vi "Send Acyclic Frame.vi"(0 "RT Data in":T1 {"End System Handle" format="%x"; "Label Transfer Config"."Block Data Refs"."Data Reference" format="%.0x"; "Status Config"."Hardware Out Dur Reference" format="%.0x"; "Status Config"."Hardware In Dur Reference" format="%.0x"; "Status Config"."Hardware Out Count Reference" format="%.0x"; "Status Config"."Hardware In Count Reference" format="%.0x"; "Status Config"."Error Data Reference" format="%.0x"; "Hardware Output Tx Channels"."Message Settings"."Transmit Channel Data Reference" format="%.0x"; "Hardware Output Tx Channels"."Message Settings"."Queue Transmit Channel" format="%.0x"; "Hardware Output Tx Channels"."Message Settings"."Driver Data"."Num Bits" min=1 max=32; "Hardware Output Tx Channels"."Message Settings"."Block Data Refs"."Data Reference" format="%.0x"; "Hardware Output Tx Channels"."Rx Com Udp Port"."Handle" format="%08x"; "Hardware Output Tx Channels"."Tx Com Udp Port"."Handle" format="%08x"; "Hardware Input Rx Channels"."Message Settings"."Transmit Channel Data Reference" format="%.0x"; "Hardware Input Rx Channels"."Message Settings"."Queue Transmit Channel" format="%.0x"; "Hardware Input Rx Channels"."Message Settings"."Driver Data"."Num Bits" min=1 max=32; "Hardware Input Rx Channels"."Message Settings"."Block Data Refs"."Data Reference" format="%.0x"; "Hardware Input Rx Channels"."Rx Com Udp Port"."Handle" format="%08x"; "Hardware Input Rx Channels"."Tx Com Udp Port"."Handle" format="%08x"}, 9 "Device Reference in":T9 format="%.0x", 11 "error in (no error)":errorcluster, 12 "Index":i32=1) -> (4 "RT Data out":T1 {"End System Handle" format="%x"; "Label Transfer Config"."Block Data Refs"."Data Reference" format="%.0x"; "Status Config"."Hardware Out Dur Reference" format="%.0x"; "Status Config"."Hardware In Dur Reference" format="%.0x"; "Status Config"."Hardware Out Count Reference" format="%.0x"; "Status Config"."Hardware In Count Reference" format="%.0x"; "Status Config"."Error Data Reference" format="%.0x"; "Hardware Output Tx Channels"."Message Settings"."Transmit Channel Data Reference" format="%.0x"; "Hardware Output Tx Channels"."Message Settings"."Queue Transmit Channel" format="%.0x"; "Hardware Output Tx Channels"."Message Settings"."Driver Data"."Num Bits" min=1 max=32; "Hardware Output Tx Channels"."Message Settings"."Block Data Refs"."Data Reference" format="%.0x"; "Hardware Output Tx Channels"."Rx Com Udp Port"."Handle" format="%08x"; "Hardware Output Tx Channels"."Tx Com Udp Port"."Handle" format="%08x"; "Hardware Input Rx Channels"."Message Settings"."Transmit Channel Data Reference" format="%.0x"; "Hardware Input Rx Channels"."Message Settings"."Queue Transmit Channel" format="%.0x"; "Hardware Input Rx Channels"."Message Settings"."Driver Data"."Num Bits" min=1 max=32; "Hardware Input Rx Channels"."Message Settings"."Block Data Refs"."Data Reference" format="%.0x"; "Hardware Input Rx Channels"."Rx Com Udp Port"."Handle" format="%08x"; "Hardware Input Rx Channels"."Tx Com Udp Port"."Handle" format="%08x"}, 15 "error out":errorcluster)   [LabVIEW 2013, in "AIT 664 Custom Device.lvlib"]
doc: "Configure com udp queued transmit hardware output channels. These channels only send when the user sets 'Transmit' high. The Transmit channel is reset to zero after the data is sent out the AIT 664 card."
uses:
  AIT 664 Custom Device.lvlib
  <vilib>/NI Veristand/Custom Device API/Custom Device Item Ref.ctl
  RT Controls/AIT 664  - RT Data.ctl
  RT Controls/AIT 664 - RT Hardware Channel.ctl
  RT Controls/AIT 664 - RT Message Settings.ctl
  <vilib>/NI Veristand/Custom Device API/Block Data Reference.ctl
  <vilib>/NI Veristand/Custom Device API/Data Reference.ctl
  RT Controls/AIT 664 - Driver Data.ctl
  Controls and Global/Start Bit.ctl
  Controls and Global/Number of Bits.ctl
  <userlib>/ARINC 664/AIT 664 Controls/General/Message Port.ctl
  <userlib>/ARINC 664/AIT 664 Controls/General/Direction.ctl
  <userlib>/ARINC 664/AIT 664 Controls/General/Message Port Type.ctl
  System Explorer/Controls/664 - Sampling Type.ctl
  RT Controls/Status Channels Config.ctl
  RT Controls/FIFO.ctl
  RT Controls/Label Transfer Config.ctl
  <vilib>/NI Veristand/Custom Device API/Data Access Type.ctl
  <vilib>/NI Veristand/Custom Device API/Global Data Refs.vi
  <vilib>/NI Veristand/Custom Device API/Custom Device API.lvlib
  <userlib>/ARINC 664/AIT 664 API.lvlib
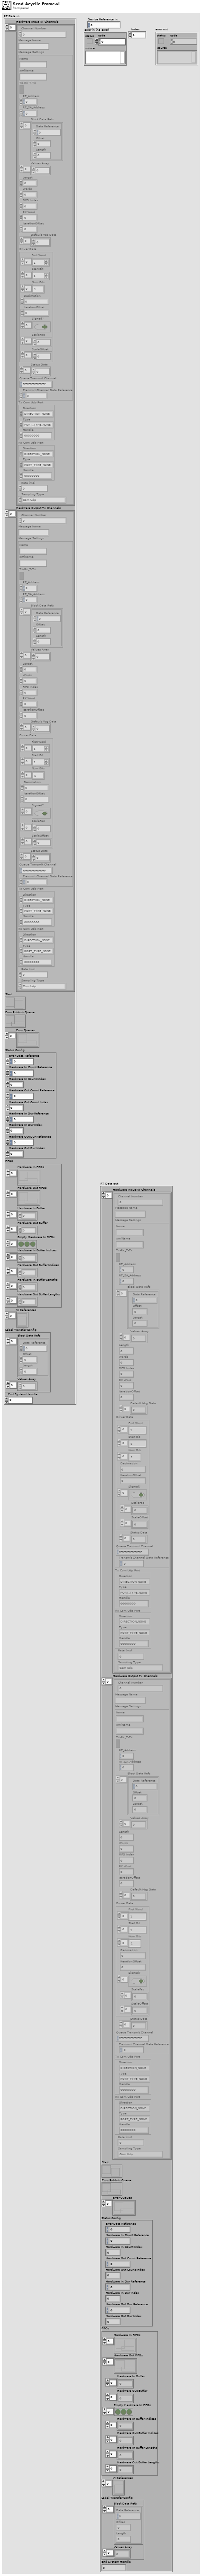
[diagram p1: front panel]
types:
  T1 = typedef "AIT 664 Custom Device.lvlib/AIT 664  - RT Data.ctl" = cluster{"Hardware Input Rx Channels":T2[], "Hardware Output Tx Channels":T2[], "Start":refnum<notifier>, "Error Publish Queue":refnum<queue>, "Error Queues":refnum<queue>[], "Status Config":T14, "FIFOs":T15, "VI References":refnum<vi>[], "Label Transfer Config":T16, "End System Handle ":u64}
  T2 = typedef "AIT 664 Custom Device.lvlib/AIT 664 - RT Hardware Channel.ctl" = cluster{"Channel Number":u16, "Message Name":string, "Message Settings":T3, "Tx Com Udp Port":T10, "Rx Com Udp Port":T10, "Rate (ms)":u32, "Sampling Type":T13}
  T3 = typedef "AIT 664 Custom Device.lvlib/AIT 664 - RT Message Settings.ctl" = cluster{"Name":string, "xmlName":string, "Tx-Rx_T-Tx":bool, "RT_Address":u8, "RT_SA_Address":u8, "Block Data Refs":T4[], "Values Array":dbl[], "Length":i32, "Words":i32, "FIFO Index":i32, "RX Word":u32, "IterationOffset":i32, "Default Msg Data":u8[], "Driver Data":T6, "Status Data":u32[], "Queue Transmit Channel":T9, "Transmit Channel Data Reference":T5}
  T4 = typedef "Custom Device API.lvlib/Block Data Reference.ctl" = cluster{"Data Reference":T5, "Offset":i32, "Length":i32}
  T5 = typedef "Custom Device API.lvlib/Data Reference.ctl" = i32
  T6 = typedef "AIT 664 Custom Device.lvlib/AIT 664 - Driver Data.ctl" = cluster{"First Word":T7[], "Start Bit":T7[], "Num Bits":T8[], "Decimation":i32, "IterationOffset":i32, "Signed?":bool[], "ScaleFac":dbl[], "ScaleOffset":dbl[]}
  T7 = typedef "AIT 664 Custom Device.lvlib/Start Bit.ctl" = i32
  T8 = typedef "AIT 664 Custom Device.lvlib/Number of Bits.ctl" = i32
  T9 = typedef "Custom Device API.lvlib/Custom Device Item Ref.ctl" = u64
  T10 = typedef "AIT 664 API.lvlib/Message Port.ctl" = cluster{"Direction":T11, "Type":T12, "Handle":u64}
  T11 = typedef "AIT 664 API.lvlib/Direction.ctl" = enum16{"DIRECTION_NONE", "DIRECTION_TX", "DIRECTION_RX"}
  T12 = typedef "AIT 664 API.lvlib/Message Port Type.ctl" = enum16{"PORT_TYPE_NONE", "COM_UDP", "SAP_UDP", "SAP_IP", "SAP_MAC", "COTS_MAC", "COTS_MAC_RAW"}
  T13 = typedef "AIT 664 Custom Device.lvlib/664 - Sampling Type.ctl" = enum16{"Com Udp", "Com Udp Queuing", "Sap Udp", "Sap Ip", "Sap Mac", "Unknown"}
  T14 = typedef "AIT 664 Custom Device.lvlib/Status Channels Config.ctl" = cluster{"Error Data Reference":T5, "Hardware In Count Reference":T5, "Hardware In Count Index":i32, "Hardware Out Count Reference":T5, "Hardware Out Count Index":i32, "Hardware In Dur Reference":T5, "Hardware In Dur Index":i32, "Hardware Out Dur Reference":T5, "Hardware Out Dur Index":i32}
  T15 = typedef "AIT 664 Custom Device.lvlib/FIFO.ctl" = cluster{"Hardware In FIFOs":refnum<k33>[], "Hardware Out FIFOs":refnum<k33>[], "Hardware In Buffer":dbl[], "Hardware Out Buffer":dbl[], "Empty Hardware In FIFOs":bool[], "Hardware In Buffer Indices":i32[], "Hardware Out Buffer Indices":i32[], "Hardware In Buffer Lengths":i32[], "Hardware Out Buffer Lengths":i32[]}
  T16 = typedef "AIT 664 Custom Device.lvlib/Label Transfer Config.ctl" = cluster{"Block Data Refs":T4[], "Values Array":dbl[]}
  T17 = typedef "Custom Device API.lvlib/Data Access Type.ctl" = enum16{"Read", "Write"}
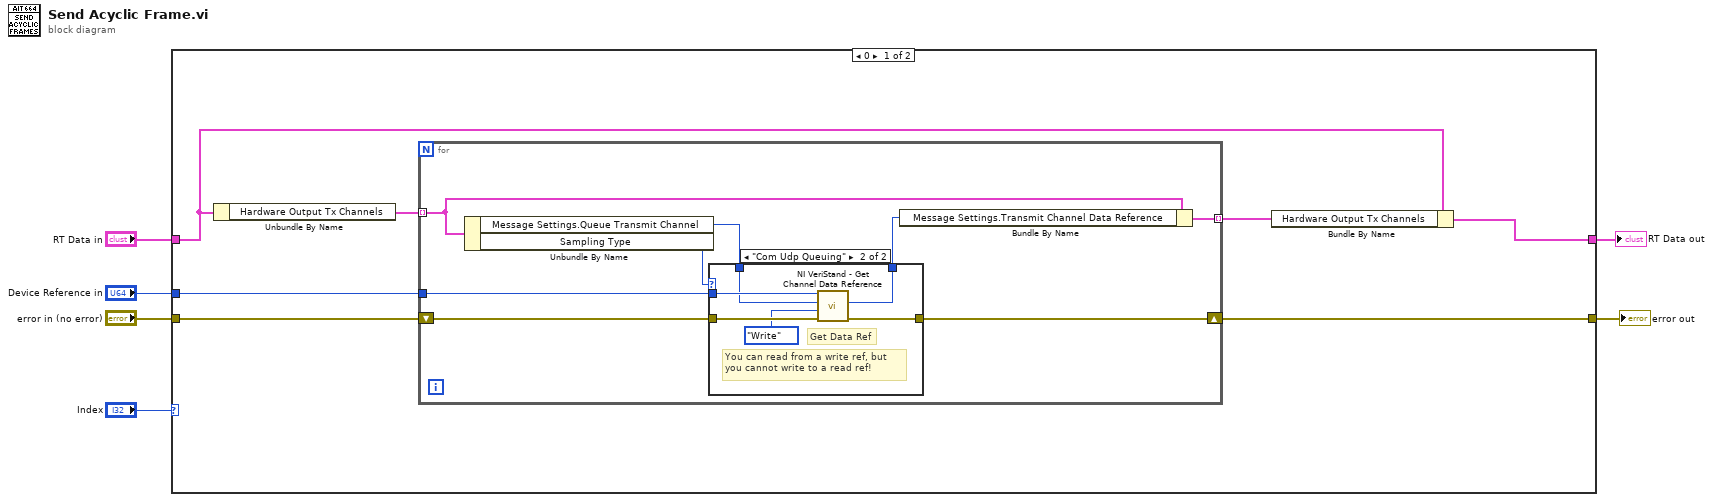
[diagram p0: block diagram]
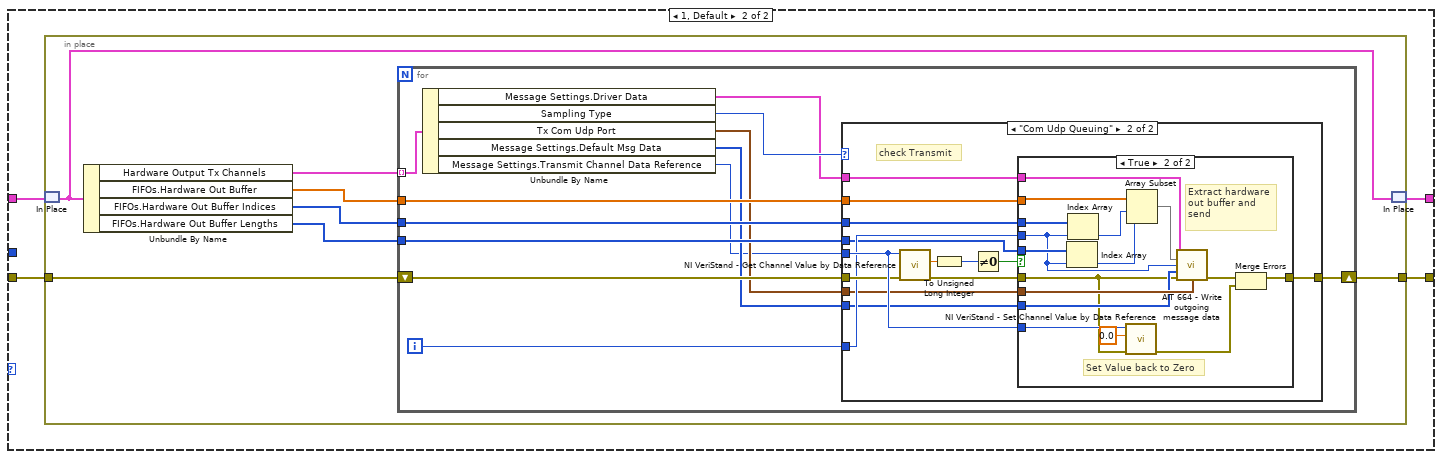
[diagram p3: hidden frame]
diagram:
  n1 = case shown="0" "Index" {
    tunnel: "error in (no error)" -> [w13 w32]
    tunnel: [w12 w31] -> w5
    tunnel: "Device Reference in" -> [w11 _]
    tunnel: "RT Data in" -> [w9 w30]
    tunnel: [w7 w29] -> w1
    frame 0 {
      n2 = Unbundle By Name(w9) -> ("Hardware Output Tx Channels"=w10:T2[])
      n3 = for {
        tunnel: w10 -> [w17] mode=indexing
        shift-right: [w18] -> w12
        shift-left: w13 -> [w21]
        tunnel: w11 -> [w20]
        tunnel: [w15] -> w8 mode=indexing
        n4 = Unbundle By Name(w17) -> ("Message Settings.Queue Transmit Channel"=w19:T9, "Sampling Type"=w14:T13)
        n5 = case shown="\"Com Udp Queuing\"" w14 {
          tunnel: w21 -> [w22 w28]
          tunnel: w20 -> [_ w27]
          tunnel: w19 -> [_ w25]
          tunnel: [w22 w24] -> w18
          tunnel: [_ w23] -> w16
          frame "Com Udp", Default {
          }
          frame "Com Udp Queuing" {
            # "You can read from a write ref, but \nyou cannot write to a read ref!"
            # "Get Data Ref"
            n6 = call <vilib>:"NI VeriStand - Get Channel Data Reference.vi"("error in (no error)"=w28, "Access"=Data_Access_Type."Write", "Channel Ref in"=w25, "Device Ref in"=w27) -> ("error out"=w24:errorcluster, "Channel Data Reference"=w23:T5)  [unwired: 5 in, 1 out]
          }
        }
        n7 = Bundle By Name(cluster=w17, "Message Settings.Transmit Channel Data Reference"=w16) -> (w15:T2)
      }
      n8 = Bundle By Name(cluster=w9, "Hardware Output Tx Channels"=w8) -> (w7:T1)
    }
    frame 1, Default {
      n9 = in-place {
        in-place-border: w32 -> [w39]
        in-place-border: [w38] -> w31
        n10 = in-place-match #1(w30) -> (w33:T1)
        n11 = Unbundle By Name(w33) -> ("Hardware Output Tx Channels"=w37:T2[], "FIFOs.Hardware Out Buffer"=w36:dbl[], "FIFOs.Hardware Out Buffer Indices"=w35:i32[], "FIFOs.Hardware Out Buffer Lengths"=w34:i32[])
        n12 = for {
          shift-right: [w51] -> w38
          shift-left: w39 -> [w50]
          tunnel: w37 -> [w49] mode=indexing
          tunnel: w36 -> [w46]
          tunnel: w35 -> [w45]
          tunnel: w34 -> [w44]
          i -> [w47]
          n13 = Unbundle By Name(w49) -> ("Message Settings.Driver Data"=w41:T6, "Sampling Type"=w48:T13, "Tx Com Udp Port"=w43:T10, "Message Settings.Default Msg Data"=w42:u8[], "Message Settings.Transmit Channel Data Reference"=w40:T5)
          n14 = case shown="\"Com Udp Queuing\"" w48 {
            tunnel: [w52 w62] -> w51
            tunnel: w40 -> [_ w61]
            tunnel: w50 -> [w52 w60]
            tunnel: w47 -> [_ w57]
            tunnel: w46 -> [_ w59]
            tunnel: w45 -> [_ w58]
            tunnel: w44 -> [_ w56]
            tunnel: w43 -> [_ w55]
            tunnel: w42 -> [_ w54]
            tunnel: w41 -> [_ w53]
            frame "Com Udp", Default {
            }
            frame "Com Udp Queuing" {
              # "check Transmit"
              n15 = call <vilib>:"NI VeriStand - Get Channel Value by Data Reference.vi"("error in (no error)"=w60, "Data Reference in"=w61) -> ("error out"=w63:errorcluster, "Value"=w66:dbl)  [unwired: 8 in]
              n16 = To Unsigned Long Integer(number=w66) -> (unsigned 32bit integer=w65:u32)
              n17 = Not Equal To 0?(x=w65) -> (x != 0?=w64:bool)
              n18 = case shown="True" w64 {
                tunnel: w63 -> [w67 w72]
                tunnel: w61 -> [_ w83]
                tunnel: [w67 w69] -> w62
                tunnel: w59 -> [_ w78]
                tunnel: w58 -> [_ w81]
                tunnel: w57 -> [_ w74]
                tunnel: w56 -> [_ w80]
                tunnel: w55 -> [_ w75]
                tunnel: w54 -> [_ w73]
                tunnel: w53 -> [_ w68]
                frame False {
                }
                frame True {
                  # "Extract hardware\nout buffer and\nsend"
                  # "Set Value back to Zero"
                  n19 = Index Array(array=w80, index=w74) -> (element=w76:i32)
                  n20 = Index Array(array=w81, index=w74) -> (element=w77:i32)
                  n21 = call <vilib>:"NI VeriStand - Set Channel Value by Data Reference.vi"("error in (no error)"=w72, "Value"=0.0, "Data Reference in"=w83) -> ("error out"=w70:errorcluster)  [unwired: 8 in]
                  n22 = Array Subset(array=w78, index=w77, length=w76) -> (w79:dbl[])
                  n23 = call "AIT 664 - Write outgoing message data.vi"("Driver Data"=w68, "Values"=w79, "Channel Index"=w74, "Msg Data In"=w73, "error in (no error)"=w72, "Tx Com Udp Port"=w75) -> ("error out"=w71:errorcluster)  [unwired: 8 in, 1 out]
                  n24 = Merge Errors(w71, w70) -> (w69:errorcluster)
                }
              }
            }
          }
        }
        n25 = in-place-match #1(w33) -> (w29:T1)
      }
    }
  }
  "error out" <- w5
  "RT Data out" <- w1
